vi "PixySigDetect.vi"(8 "error in (no error)":errorcluster, 10 "Signature Number":u8, 11 "VISA resource name":refnum<visa-resource-name>) -> (0 "error out":errorcluster, 1 "Data":string, 2 "Detected":bool, 3 "VISA resource name out":refnum<visa-resource-name>)   [LabVIEW 2017]
panel:
  out "Serial Command":string
  out "Raw Input":string
  out "Data Length":u8
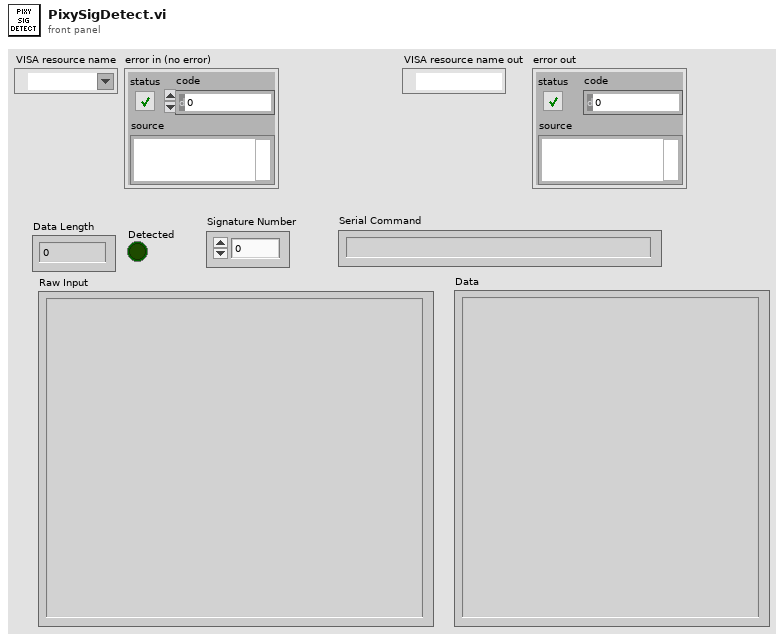
[diagram p1: front panel]
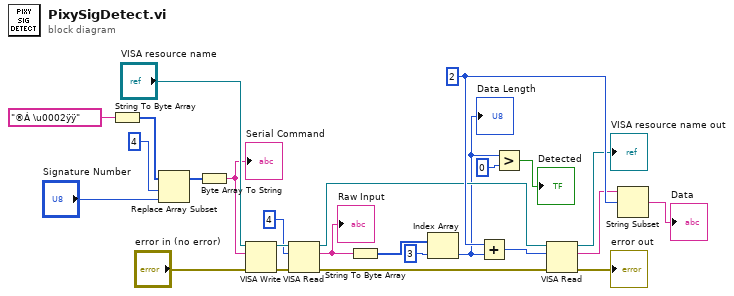
[diagram p0: block diagram]
diagram:
  w23 = u8 2 ("x")
  n1 = String To Byte Array(string="®Á \u0002ÿÿ") -> (unsigned byte array=w5:u8[])
  n2 = Replace Array Subset(array=w5, new element="Signature Number", index=4) -> (w2:u8[])
  n3 = Byte Array To String(unsigned byte array=w2) -> (string=w1:string)
  "Serial Command" <- w1
  n4 = VISA Write(VISA resource name="VISA resource name", write buffer=w1, error in (no error)="error in (no error)") -> (VISA resource name out=w21:refnum<visa-resource-name>, error out=w22:errorcluster)  [unwired: 1 out]
  n5 = VISA Read(VISA resource name=w21, byte count=u32 4 ("Character Count"), error in (no error)=w22) -> (VISA resource name out=w16:refnum<visa-resource-name>, read buffer=w19:string, error out=w15:errorcluster)  [unwired: 1 out]
  "Raw Input" <- w19
  n6 = String To Byte Array(string=w19) -> (unsigned byte array=w24:u8[])
  n7 = Index Array(array=w24, index=3) -> (element=w10:u8)
  "Data Length" <- w10
  n8 = Add(x=w23, y=w10) -> (x+y=w17:u8)
  n9 = Greater?(x=w10, y=u8 0) -> (0:→"Detected":bool)
  n10 = VISA Read(VISA resource name=w16, byte count=w17, error in (no error)=w15) -> (VISA resource name out=→"VISA resource name out":refnum<visa-resource-name>, read buffer=w18:string, error out=→"error out":errorcluster)  [unwired: 1 out]
  n11 = String Subset(string=w18, offset (0)=w23) -> (substring=→"Data":string)  [unwired: 1 in]
